vi "Trav_Axis_Correction.vi"(0 "Traverse Name":string, 1 "Axis":T1, 2 "Position input XYZ":sgl[](array[numeric])=[0.0, 0.0, 0.0] format="%.2f") -> (3 "Position":dbl[](array[numeric]), 4 "Correction":dbl[](array[numeric]), 5 "Offset Array":sgl[](array[numeric]), 6 "Error String":string)   [LabVIEW 2022 SP3]
uses:
  Route mapping/Axis.ctl
  Globals/Constants_global.vi
panel:
  out "fractional index or x":dbl
  out "In Range?":bool
  out "Data Found?":bool
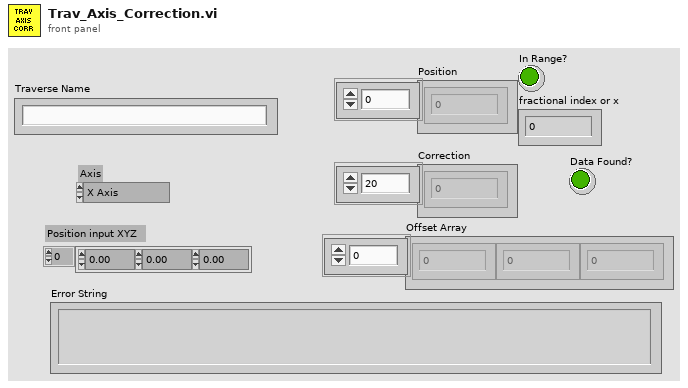
[diagram p1: front panel]
types:
  T1 = typedef "Axis.ctl" = enum16{"X Axis", "X Axis -ve", "Y Axis", "Y Axis -ve", "Z Axis", "Z Axis -ve"}
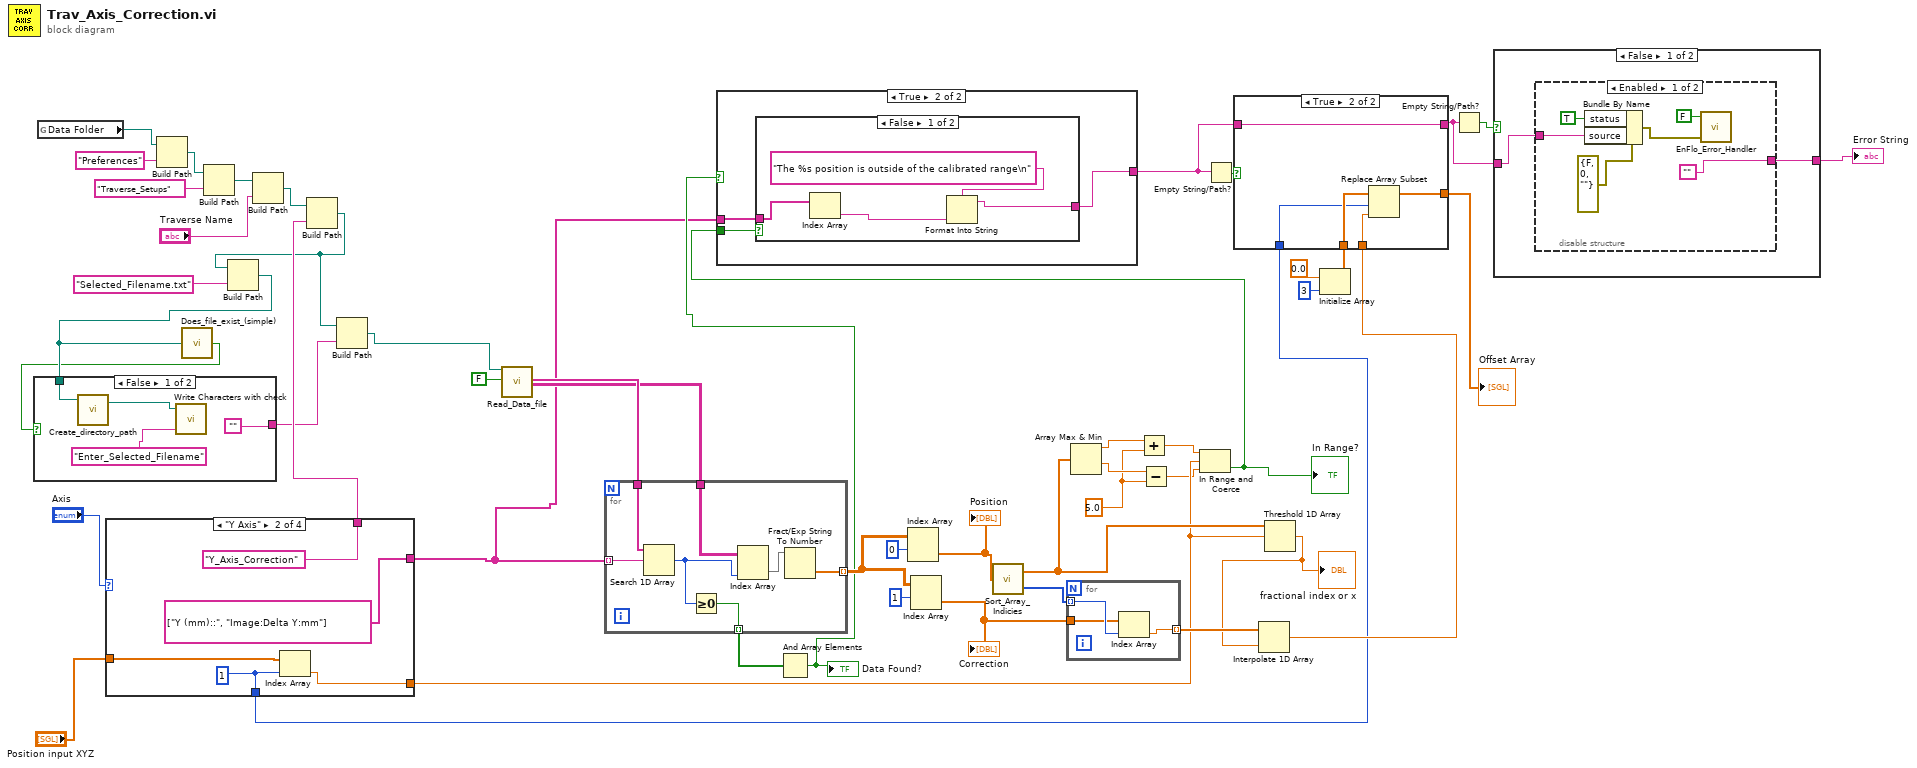
[diagram p0: block diagram]
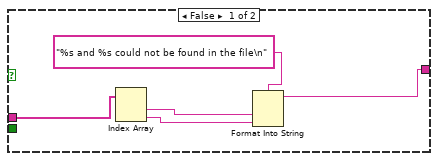
[diagram p2: hidden frame]
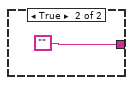
[diagram p3: hidden frame]
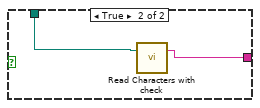
[diagram p6: hidden frame]
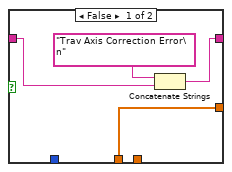
[diagram p7: hidden frame]
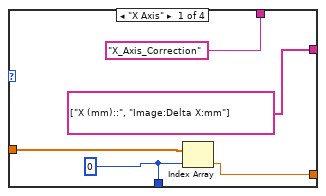
[diagram p8: hidden frame]
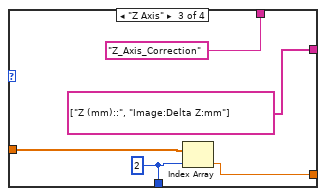
[diagram p9: hidden frame]
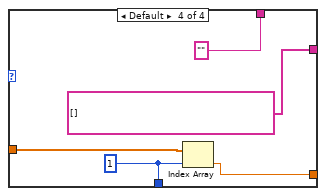
[diagram p10: hidden frame]
diagram:
  w27 = 5.0 ("y")
  n1 = global read "Constants_global.vi" "Data Folder"() -> (w48:path)
  n2 = case shown="\"Y Axis\"" "Axis" {
    tunnel: ["X_Axis_Correction" ("name or relative path") "Y_Axis_Correction" ("name or relative path") "Z_Axis_Correction" ("name or relative path") "" ("name or relative path")] -> w10
    tunnel: [string[] ["X (mm)::", "Image:Delta X:mm"] ("Ch names Out") string[] ["Y (mm)::", "Image:Delta Y:mm"] ("Ch names Out") string[] ["Z (mm)::", "Image:Delta Z:mm"] ("Ch names Out") string[] [] ("Ch names Out")] -> w21
    tunnel: "Position input XYZ" -> [w52 w57 w62 w67]
    tunnel: [w51 w56 w61 w66] -> w26
    tunnel: [w50 w55 w60 w65] -> w13
    frame "X Axis" {
      w50 = 0 ("index")
      n3 = Index Array(array=w52, index=w50) -> (element=w51:sgl)
    }
    frame "Y Axis" {
      w55 = 1 ("index")
      n4 = Index Array(array=w57, index=w55) -> (element=w56:sgl)
    }
    frame "Z Axis" {
      w60 = 2 ("index")
      n5 = Index Array(array=w62, index=w60) -> (element=w61:sgl)
    }
    frame Default {
      w65 = 1 ("index")
      n6 = Index Array(array=w67, index=w65) -> (element=w66:sgl)
    }
  }
  n7 = Build Path(base path=w48, name or relative path="Preferences") -> (appended path=w46:path)
  n8 = Build Path(base path=w46, name or relative path="Traverse_Setups") -> (appended path=w45:path)
  n9 = Build Path(base path=w45, name or relative path="Traverse Name") -> (appended path=w11:path)
  n10 = Build Path(base path=w11, name or relative path=w10) -> (appended path=w9:path)
  n11 = Build Path(base path=w9, name or relative path="Selected_Filename.txt" ("Substring")) -> (appended path=w7:path)
  n12 = call "Does_file_exist_(simple).vi"("Pathname"=w7) -> ("exists?"=w6:bool)
  n13 = case shown="False" w6 {
    tunnel: w7 -> [w73 w75]
    tunnel: ["" w74] -> w5
    frame False {
      n14 = call "Create_directory_path.vi"("Path name"=w73) -> ("Path name Out"=w71:path)  [unwired: 2 in, 1 out]
      n15 = call "Write Characters with check.vi"("String to Write"="Enter_Selected_Filename" ("Substring"), "file (use dialog)"=w71) -> ()  [unwired: 2 in, 1 out]
    }
    frame True {
      n16 = call "Read Characters with check.vi"("file (use dialog)"=w75) -> ("Read String"=w74:string)  [unwired: 1 in, 1 out]
    }
  }
  n17 = Build Path(base path=w9, name or relative path=w5) -> (appended path=w8:path)
  n18 = call "Read_Data_file.vi"("Results file"=w8, "Delete First Rows?"=FALSE) -> ("Ch names Out"=w43:string[], "Channel Values Out"=w42:string[][])  [unwired: 5 in, 11 out]
  n19 = for {
    tunnel: w43 -> [w82]
    tunnel: w21 -> [w81] mode=indexing
    tunnel: w42 -> [w80]
    tunnel: [w79] -> w39 mode=indexing
    tunnel: [w76] -> w38 mode=indexing
    n20 = Search 1D Array(1D array=w82, element=w81) -> (index of element=w77:i32)  [unwired: 1 in]
    n21 = Greater Or Equal To 0?(x=w77) -> (x >= 0?=w76:bool)
    n22 = Index Array(array=w80, index (col)=w77) -> (element=w78:string[])  [unwired: 1 in]
    n23 = Fract/Exp String To Number(string=w78) -> (number=w79:dbl[])  [unwired: 3 in, 1 out]
  }
  n24 = And Array Elements(Boolean array=w38) -> (logical AND=w22:bool)
  "Data Found?" <- w22
  n25 = Index Array(array=w39, index (row)=0) -> (element=w35:dbl[])  [unwired: 1 in]
  "Position" <- w35
  n26 = Index Array(array=w39, index (row)=1) -> (element=w33:dbl[])  [unwired: 1 in]
  "Correction" <- w33
  n27 = call "Sort_Array_Indicies.vi"("unsorted array"=w35) -> ("sorted array"=w30:dbl[], "Sort Index"=w34:i32[])
  n28 = for {
    tunnel: w34 -> [w85] mode=indexing
    tunnel: w33 -> [w84]
    tunnel: [w83] -> w32 mode=indexing
    n29 = Index Array(array=w84, index=w85) -> (element=w83:dbl)
  }
  n30 = Array Max & Min(array=w30) -> (max value=w29:dbl, min value=w28:dbl)  [unwired: 2 out]
  n31 = Add(x=w29, y=w27) -> (x+y=w25:dbl)
  n32 = Subtract(x=w28, y=w27) -> (x-y=w24:dbl)
  n33 = In Range and Coerce(upper limit=w25, x=w26, lower limit=w24) -> (In Range?=w23:bool)  [unwired: 1 out]
  "In Range?" <- w23
  n34 = case shown="True" w22 {
    tunnel: w23 -> [_ w93]
    tunnel: [w86 w92] -> w19
    tunnel: w21 -> [w89 w91]
    frame False {
      n35 = Index Array(array=w89) -> (element #1=w90:string, element #2=w88:string)  [unwired: 2 in]
      n36 = Format Into String(format string="%s and %s could not be found in the file\n", w90, w88) -> (resulting string=w86:string)  [unwired: 2 in, 1 out]
    }
    frame True {
      n37 = case shown="False" w93 {
        tunnel: w91 -> [w96 _]
        tunnel: [w94 ""] -> w92
        frame False {
          n38 = Index Array(array=w96) -> (element=w95:string)  [unwired: 1 in]
          n39 = Format Into String(format string="The %s position is outside of the calibrated range\n", w95) -> (resulting string=w94:string)  [unwired: 2 in, 1 out]
        }
        frame True {
        }
      }
    }
  }
  n40 = Empty String/Path?(string/path=w19) -> (empty?=w20:bool)
  n41 = Threshold 1D Array(2:w26, 3:w30) -> (0:w31:dbl)  [unwired: 1 in]
  "fractional index or x" <- w31
  n42 = Interpolate 1D Array(1:w31, 2:w32) -> (0:w18:dbl)
  n43 = Initialize Array(sgl 0.0, 3 ("dimension size")) -> (w15:sgl[])
  n44 = case shown="True" w20 {
    tunnel: [w100 w107] -> w2
    tunnel: w19 -> [w102 w107]
    tunnel: w18 -> [_ w106]
    tunnel: w15 -> [w99 w105]
    tunnel: [w99 w104] -> w14
    tunnel: w13 -> [_ w103]
    frame False {
      n45 = Concatenate Strings("Trav Axis Correction Error\n" ("string"), w102) -> (w100:string)
    }
    frame True {
      n46 = Replace Array Subset(array=w105, new element=w106, index=w103) -> (w104:sgl[])
    }
  }
  "Offset Array" <- w14
  n47 = Empty String/Path?(string/path=w2) -> (empty?=w4:bool)
  n48 = case shown="False" w4 {
    tunnel: [w108 w117] -> w3
    tunnel: w2 -> [w109 w117]
    frame False {
      n49 = disable-structure shown="Enabled" {
        disable-tunnel: w109 -> [w115 w116]
        disable-tunnel: ["" w116] -> w108
        frame Enabled {
          n50 = Bundle By Name(cluster=errorcluster {"status"=FALSE, "code"=0, "source"=""} ("error in (no error)"), "status"=TRUE, "source"=w115) -> (w111:errorcluster)
          n51 = call "EnFlo_Error_Handler.vi"("error in (no error)"=w111, "Dialog Box (F)"=FALSE ("Dialog Box (T)")) -> ()  [unwired: 2 in, 2 out]
        }
        frame Disabled {
        }
      }
    }
    frame True {
    }
  }
  "Error String" <- w3
